vi "Submit request array.vi"(7 "Server Address":string, 8 "error in (no error)":errorcluster, 10 "Request Array":string[](array[string])) -> (0 "error out":errorcluster, 1 "body":string, 2 "Return Data Array":string[](array[string]))   [LabVIEW 2018, in "Collaborator.lvlib"]
uses:
  Collaborator.lvlib
  e0056f21-56ba-414d-8bd7-9d7eed923aa9.vi
  <vilib>/httpClient/POSTBuffer.vi
  <vilib>/JDP Science/JSONtext/JSON text to Variant.vi
  <vilib>/httpClient/LabVIEWHTTPClient.lvlib
  <vilib>/JDP Science/JSONtext/JSONtext.lvlib
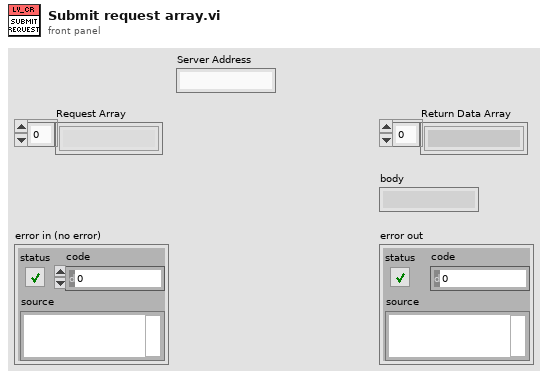
[diagram p1: front panel]
types:
  T1 = typedef "LabVIEWHTTPClient.lvlib/ClientHandle.ctl" = refnum<k1>
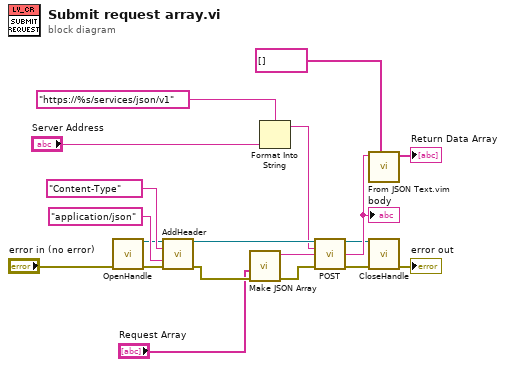
[diagram p0: block diagram]
diagram:
  n1 = call <vilib>:"OpenHandle.vi"("error in (no error)"="error in (no error)") -> ("client handle out"=w8:T1, "error out"=w5:errorcluster)  [unwired: 13 in]
  n2 = call <vilib>:"AddHeader.vi"("client handle"=w8, "header"="Content-Type", "value"="application/json", "error in (no error)"=w5) -> ("client handle out"=w9:T1, "error out"=w17:errorcluster)  [unwired: 10 in]
  n3 = call <vilib>:"Make JSON Array.vi"("error in (no error)"=w17, "JSON Elements"="Request Array") -> ("error out"=w18:errorcluster, "<JSON>"=w16:string)  [unwired: 8 in]
  n4 = Format Into String(format string="https://%s/services/json/v1" ("url"), "Server Address") -> (resulting string=w1:string)  [unwired: 2 in, 1 out]
  n5 = call-poly <vilib>:"POST.vi"("client handle"=w9, "url"=w1, "buffer"=w16, "error in (no error)"=w18) -> ("client handle out"=w4:T1, "body"=w12:string, "error out"=w6:errorcluster)  [unwired: 8 in, 1 out]
  "body" <- w12
  n6 = call "From JSON Text.vim"("Data Type and Default Value"=string[] [], "JSON"=w12) -> ("Data out"=→"Return Data Array":string[])  [unwired: 8 in, 1 out]
  n7 = call <vilib>:"CloseHandle.vi"("client handle"=w4, "error in (no error)"=w6) -> ("error out"=→"error out":errorcluster)  [unwired: 13 in]
